vi "Cliente-ServidorFullDuplex.vi"() -> ()   [LabVIEW 2019]
uses:
  <vilib>/Instr/_visa.llb/VISA Configure Serial Port (Instr).vi
panel:
  out "String":string
  in  "stop":bool
  in  "Baudios DAQ":T1(ring)
  in  "Conectar Puerto\nRS232":refnum<visa-resource-name>
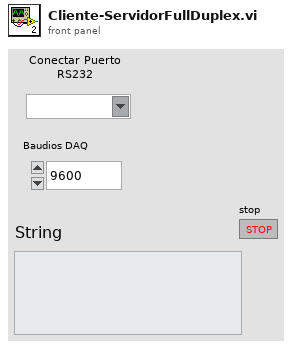
[diagram p1: front panel]
types:
  T1 = enum16{"9600", "14400", "19200", "38400", "56000", "57600", "115200"}
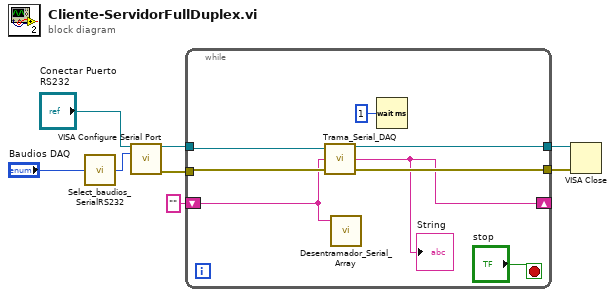
[diagram p0: block diagram]
diagram:
  n1 = call "Select_baudios_SerialRS232.vi"("Baudios"="Baudios DAQ") -> ("baud rate (9600)"=w7:u32)
  n2 = call-poly "VISA Configure Serial Port"("VISA resource name"="Conectar Puerto\nRS232", "baud rate (9600)"=w7) -> ("VISA resource name out"=w5:refnum<visa-resource-name>, "error out"=w4:errorcluster)  [unwired: 12 in]
  n3 = while {
    tunnel: w5 -> [w16]
    tunnel: w4 -> [w15]
    tunnel: [w14] -> w3
    tunnel: [w13] -> w2
    shift-right: [w9] -> _
    shift-left: "" ("name (unnamed)") -> [w10]
    stop <- "stop" stop-if-true
    n4 = call "Trama_Serial_DAQ.vi"("error in (no error)"=w15, "memoria_trama"=w10, "reference"=w16) -> ("error out"=w13:errorcluster, "Trama_Out"=w9:string, "reference 2"=w14:refnum<visa-resource-name>)
    "String" <- w9
    n5 = call "Desentramador_Serial_Array.vi"("Trama_Serial"=w10) -> ()  [unwired: 6 in, 1 out]
    n6 = Wait (ms)(milliseconds to wait=u32 1) -> ()  [unwired: 1 out]
  }
  n7 = VISA Close(VISA resource name=w3, error in (no error)=w2) -> ()  [unwired: 1 out]
